vi "get_signal_list.vi"(1 "Refnum in":refnum<k21>) -> (0 "Sigs":refnum<k21>[](array[refnum]))   [LabVIEW 2017]
uses:
  <resource>/objmgr/xnet.rc
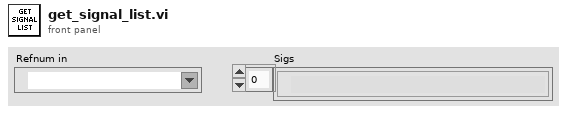
[diagram p1: front panel]
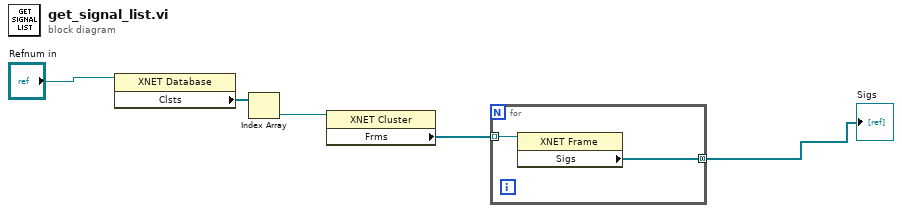
[diagram p0: block diagram]
diagram:
  n1 = property class="XNET Database"(reference="Refnum in") -> ("Clsts"=w2:refnum<k21>[])  [unwired: 1 in, 2 out]
  n2 = Index Array(array=w2) -> (element=w3:refnum<k21>)  [unwired: 1 in]
  n3 = property class="XNET Cluster"(reference=w3) -> ("Frms"=w4:refnum<k21>[])  [unwired: 1 in, 2 out]
  n4 = for {
    tunnel: [w7] -> w5 mode=concatenating
    tunnel: w4 -> [w6] mode=indexing
    n5 = property class="XNET Frame"(reference=w6) -> ("Sigs"=w7:refnum<k21>[])  [unwired: 1 in, 2 out]
  }
  "Sigs" <- w5
